vi "example-InsertMenuItemsWithShortcut.vi"() -> ()   [LabVIEW 2021]
uses:
  a1b5153a-e3ee-49e1-af71-bc127d6ac68d.vi
  <vilib>/Comparison/Equal/Equal Functor/Equal Functor.lvclass
panel:
  in  "String":string
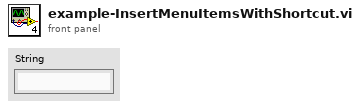
[diagram p1: front panel]
types:
  T1 = cluster{"Name":string, "Include Shift Key?":bool, "Include Ctrl Key?":bool, "Shortcut Key":string}[]
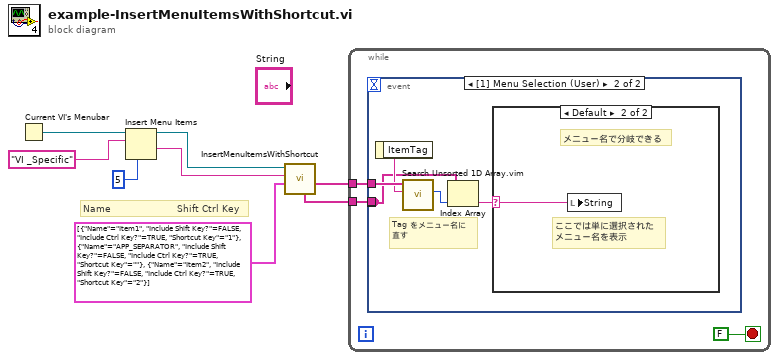
[diagram p0: block diagram]
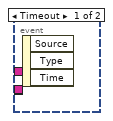
[diagram p2: hidden frame]
diagram:
  # "Name                      Shift Ctrl Key"
  n1 = Current VI's Menubar() -> (w8:refnum<k9>)
  n2 = Insert Menu Items(4:5 ("Insert After (last)"), 8:"VI _Specific" ("Menu Name"), 9:w8) -> (1:w1:string, 3:w4:refnum<k9>)  [unwired: 3 in, 1 out]
  n3 = call "InsertMenuItemsWithShortcut.vi"("Sub Items"=T1 [{"Name"="Item1", "Include Shift Key?"=FALSE, "Include Ctrl Key?"=TRUE, "Shortcut Key"="1"}, {"Name"="APP_SEPARATOR", "Include Shift Key?"=FALSE, "Include Ctrl Key?"=TRUE, "Shortcut Key"=""}, {"Name"="Item2", "Include Shift Key?"=FALSE, "Include Ctrl Key?"=TRUE, "Shortcut Key"="2"}], "Target Tag"=w1, "menu ref"=w4) -> ("Sub Item Tags"=w6:string[], "Sub Item Names"=w5:string[])  [unwired: 5 in, 2 out]
  n4 = while {
    tunnel: w6 -> [w10]
    tunnel: w5 -> [w9]
    stop <- FALSE stop-if-true
    n5 = event shown="[1] Menu Selection (User)" {
      selector: _ -> [_ _]
      dyn-events: _ -> [_ _]
      timeout: _ -> [_ _]
      tunnel: w10 -> [_ w16]
      tunnel: [_ w14] -> _
      tunnel: w9 -> [_ w14]
      event Timeout {
        n6 = event-data() -> ()  [unwired: 1 in, 3 out]
      }
      event Menu Selection (User) {
        # "Tag をメニュー名に\n直す"
        n7 = event-data() -> ("ItemTag"=w15:string)  [unwired: 1 in]
        n8 = call "Search Unsorted 1D Array.vim"("element"=w15, "unsorted 1D array"=w16) -> ("index of element"=w13:i32)  [unwired: 9 in]
        n9 = Index Array(array=w14, index=w13) -> (element=w12:string)
        n10 = case shown="Default" w12 {
          selector: w12 -> [_ w17]
          frame "" {
          }
          frame Default {
            # "ここでは単に選択された\nメニュー名を表示"
            # "メニュー名で分岐できる"
            n11 = local write "String"(w17) -> ()
          }
        }
      }
    }
  }
